vi "DAQmx Read (Power 2D I16 NChan NSamp).vi"(0 "task/channels in":refnum<k21>, 7 "number of samples per channel":i32=-1, 9 "timeout":dbl=10.0 format="%0.2f", 11 "error in":errorcluster) -> (4 "task out":refnum<k21>, 6 "voltage":i16[][](array[numeric]), 8 "current":i16[][](array[numeric]), 15 "error out":errorcluster)   [LabVIEW 2022 SP3]
doc: "Reads one or more unscaled 16-bit signed integer samples from a task that contains one or more power channels."
uses:
  nilvaiu.dll
panel:
  # "channel"
  # "sample #"
  # "channel"
  # "sample #"
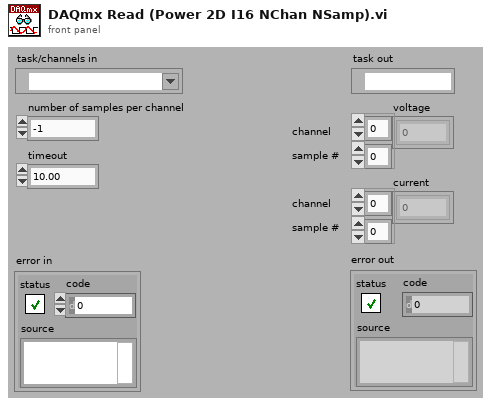
[diagram p1: front panel]
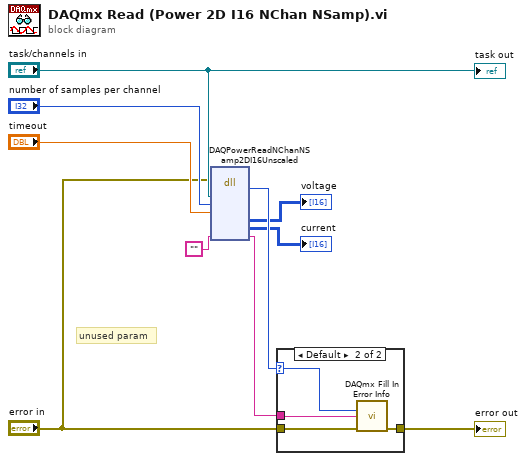
[diagram p0: block diagram]
diagram:
  # "unused param"
  n1 = dll-call lib="nilvaiu.*" fn="DAQPowerReadNChanNSamp2DI16Unscaled"(error in="error in", "taskID"="task/channels in", "numberOfSamples"="number of samples per channel", "timeout"="timeout", "extendedErrorInfo"="") -> ("return type"=w8:i32, "voltage"=→"voltage":i16[][], "current"=→"current":i16[][], "extendedErrorInfo"=w5:string)  [unwired: 5 in, 4 out]
  n2 = case shown="Default" w8 {
    selector: w8 -> [_ w13]
    tunnel: "error in" -> [w11 w15]
    tunnel: [w11 w14] -> w10
    tunnel: w5 -> [_ w12]
    frame 0 {
    }
    frame Default {
      n3 = call "DAQmx Fill In Error Info.vi"("status code"=w13, "extended error info"=w12, "error in"=w15) -> ("error out"=w14:errorcluster)  [unwired: 1 in, 11 out]
    }
  }
  "error out" <- w10
  "task out" <- "task/channels in"
